vi "Update Limit On Off.vi"(0 "Notifier Name":string, 7 "Use Limits?":bool, 11 "Error In":errorcluster) -> (15 "Error Out":errorcluster)   [LabVIEW 2020]
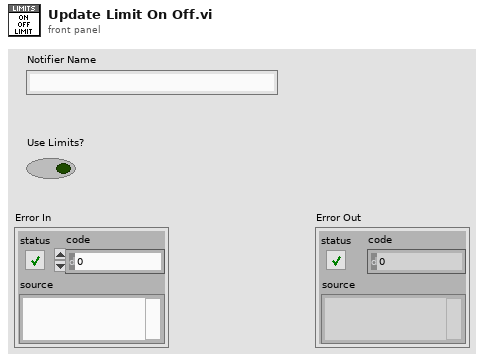
[diagram p1: front panel]
types:
  T1 = typedef "Stage Limits.ctl" = cluster{"Notifier":string, "Use Limits":bool, "Limits":dbl[][]}
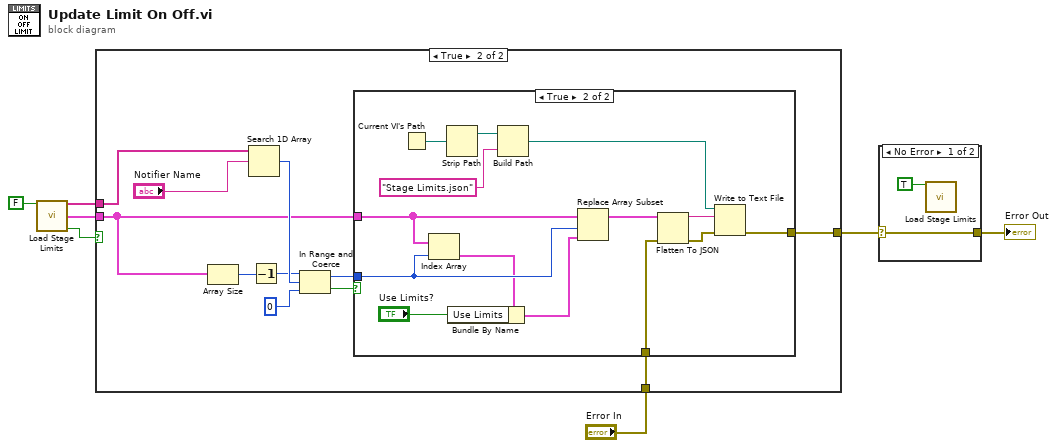
[diagram p0: block diagram]
diagram:
  n1 = call "Load Stage Limits.vi"("Update Limits"=FALSE) -> ("Notifier Names"=w6:string[], "Stage Limits"=w5:T1[], "Loaded"=w4:bool)  [unwired: 12 in]
  n2 = case shown="True" w4 {
    tunnel: w6 -> [_ w19]
    tunnel: w5 -> [_ w12]
    tunnel: [w8 w10] -> w3
    tunnel: "Error In" -> [w8 w9]
    frame False {
    }
    frame True {
      n3 = Array Size(array=w12) -> (size(s)=w16:i32)
      n4 = Search 1D Array(1D array=w19, element="Notifier Name") -> (index of element=w17:i32)  [unwired: 1 in]
      n5 = Decrement(x=w16) -> (x-1=w15:i32)
      n6 = In Range and Coerce(upper limit=w15, x=w17, lower limit=0) -> (coerced(x)=w13:i32, In Range?=w14:bool)
      n7 = case shown="True" w14 {
        tunnel: w13 -> [_ w22]
        tunnel: w12 -> [_ w23]
        tunnel: [w20 w25] -> w10
        tunnel: w9 -> [w20 w24]
        frame False {
        }
        frame True {
          n8 = Current VI's Path() -> (path=w29:path)
          n9 = Index Array(array=w23, index=w22) -> (element=w21:T1)
          n10 = Strip Path(path=w29) -> (stripped path=w28:path)  [unwired: 1 out]
          n11 = Bundle By Name(cluster=w21, "Use Limits"="Use Limits?") -> (w34:T1)
          n12 = Build Path(base path=w28, name or relative path="Stage Limits.json") -> (appended path=w26:path)
          n13 = Replace Array Subset(array=w23, new element=w34, index=w22) -> (w31:T1[])
          n14 = Flatten To JSON(anything=w31, error in (no error)=w24) -> (JSON string=w32:string, 11:w30:errorcluster)  [unwired: 1 in]
          n15 = Write to Text File(file (use dialog)=w26, text=w32, error in=w30) -> (error out=w25:errorcluster)  [unwired: 1 in, 2 out]
        }
      }
    }
  }
  n16 = case shown="No Error" w3 {
    selector: w3 -> [w35 w37]
    tunnel: [w35 w37] -> w2
    frame No Error {
      n17 = call "Load Stage Limits.vi"("Update Limits"=TRUE) -> ()  [unwired: 12 in, 3 out]
    }
    frame Error {
    }
  }
  "Error Out" <- w2
